vi "PhotonPoseEstimator_multiTagOnCoprocStrategy.vi"(10 "CameraResult":T11, 11 "PhotonPoseEstimator_REF":T1) -> (0 "Do Alt Strategy":bool, 1 "Pos Found":bool, 3 "PhotonEstimatedRobotPose":T2={"EstimatedPose"={"Translation3d"={"X"=0.0, "Y"=0.0, "Z"=0.0}, "Rotation3d"={"Q_quaternion"={"R"=1.0, "V"=[0.0, 0.0, 0.0]}}}, "TimeStamp_Seconds"=0.0, "targetsUsed"=[], "Strategy"=enum."LOWEST_AMBIGUITY"} {"targetsUsed"."AltCameraToTarget"."TRANSLATION3D"."Z" format="%14.3f"; "targetsUsed"."AltCameraToTarget"."TRANSLATION3D"."Y" format="%14.3f"; "targetsUsed"."AltCameraToTarget"."TRANSLATION3D"."X" format="%14.3f"; "targetsUsed"."BestCameraToTarget"."TRANSLATION3D"."Z" format="%14.3f"; "targetsUsed"."BestCameraToTarget"."TRANSLATION3D"."Y" format="%14.3f"; "targetsUsed"."BestCameraToTarget"."TRANSLATION3D"."X" format="%14.3f"; "EstimatedPose"."Translation3d"."Z" format="%14.3f"; "EstimatedPose"."Translation3d"."Y" format="%14.3f"; "EstimatedPose"."Translation3d"."X" format="%14.3f"})   [LabVIEW 2019, in "PhotonVisionLib.lvlib"]
doc: "This is an internal function. Use Update or Update_Pipeline instead of this function.\n\nDetermine the best target based the multi-target routine on the coprocessor"
uses:
  PhotonVisionLib.lvlib
  Enum/PhotonPoseStrategy_ENUM.ctl
  <vilib>/Rock Robotics/WPI/ThirdParty/JAS_Junk/TrajLib/Trajectory_Library.lvlib
  <vilib>/Rock Robotics/WPI/ThirdParty/JAS_Junk/TrajLib/TypeDef/TRANSLATION3D.ctl
  <vilib>/Rock Robotics/WPI/ThirdParty/JAS_Junk/TrajLib/TypeDef/QUATERNION.ctl
  <vilib>/Rock Robotics/WPI/ThirdParty/JAS_Junk/TrajLib/TypeDef/ROTATION3D.ctl
  <vilib>/Rock Robotics/WPI/ThirdParty/JAS_Junk/TrajLib/TypeDef/TRANSFORM3D.ctl
  <vilib>/Rock Robotics/WPI/ThirdParty/JAS_Junk/TrajLib/TypeDef/POSE3D.ctl
  TypeDef/PhotonEstimatedRobotPoseType.ctl
  TypeDef/TargetCornerType.ctl
  TypeDef/PhotonTrackedTargetType.ctl
  TypeDef/PhotonPipelineResultType.ctl
  <vilib>/Rock Robotics/WPI/ThirdParty/JAS_Junk/TrajLib/TypeDef/AprilTag.ctl
  <vilib>/Rock Robotics/WPI/ThirdParty/JAS_Junk/TrajLib/Enum/AprilTagFieldLayoutOrignPosition_ENUM.ctl
  <vilib>/Rock Robotics/WPI/ThirdParty/JAS_Junk/TrajLib/TypeDef/AprilTagFieldLayout.ctl
  TypeDef/PhotonPoseEstimatorType.ctl
  TypeDef/PhotonPNPResultType.ctl
  TypeDef/PhotonMultiTargetPNPResultType.ctl
  TypeDef/PhotonTargetModel.ctl
  Ref/PhotonPipelineResult_REF.ctl
  Ref/PhotonPoseEstimator_REF.ctl
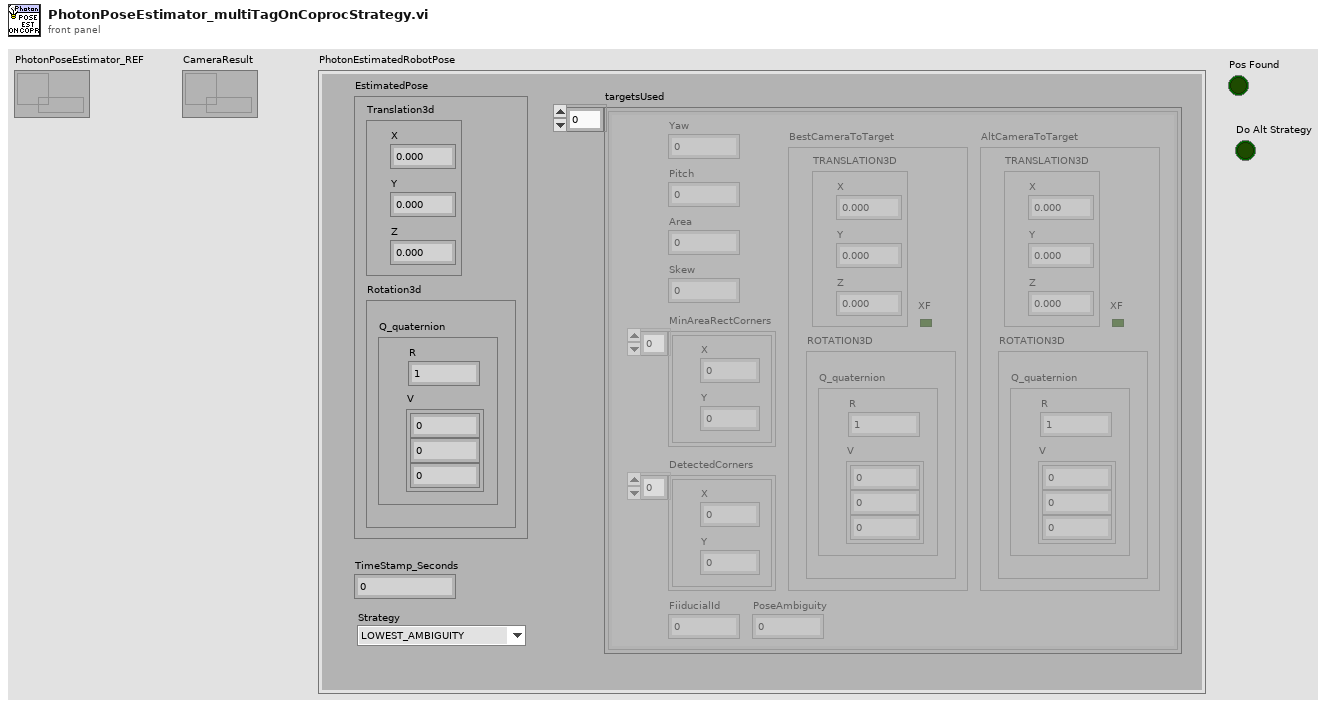
[diagram p1: front panel]
types:
  T1 = typedef "PhotonVisionLib.lvlib/PhotonPoseEstimator_REF.ctl" = refnum<data-value>
  T2 = typedef "PhotonVisionLib.lvlib/PhotonEstimatedRobotPoseType.ctl" = cluster{"EstimatedPose":T3, "TimeStamp_Seconds":dbl, "targetsUsed":T7[], "Strategy":T10}
  T3 = typedef "Trajectory_Library.lvlib/POSE3D.ctl" = cluster{"Translation3d":T4, "Rotation3d":T5}
  T4 = typedef "Trajectory_Library.lvlib/TRANSLATION3D.ctl" = cluster{"X":dbl, "Y":dbl, "Z":dbl}
  T5 = typedef "Trajectory_Library.lvlib/ROTATION3D.ctl" = cluster{"Q_quaternion":T6}
  T6 = typedef "Trajectory_Library.lvlib/QUATERNION.ctl" = cluster{"R":dbl, "V":dbl[]}
  T7 = typedef "PhotonVisionLib.lvlib/PhotonTrackedTargetType.ctl" = cluster{"Yaw":dbl, "Pitch":dbl, "Area":dbl, "Skew":dbl, "MinAreaRectCorners":T8[], "BestCameraToTarget":T9, "FiiducialId":i32, "AltCameraToTarget":T9, "PoseAmbiguity":dbl, "DetectedCorners":T8[]}
  T8 = typedef "PhotonVisionLib.lvlib/TargetCornerType.ctl" = cluster{"X":dbl, "Y":dbl}
  T9 = typedef "Trajectory_Library.lvlib/TRANSFORM3D.ctl" = cluster{"TRANSLATION3D":T4, "ROTATION3D":T5, "XF":bool}
  T10 = typedef "PhotonVisionLib.lvlib/PhotonPoseStrategy_ENUM.ctl" = enum16{"LOWEST_AMBIGUITY", "CLOSEST_TO_CAMERA_HEIGHT", "CLOSEST_TO_REFERENCE_POSE", "CLOSEST_TO_LAST_POSE", "AVERAGE_BEST_TARGETS", "MULTI_TAG_PNP_ON_COPROCESSOR", "MULTI_TAG_PNP_ON_RIO"}
  T11 = typedef "PhotonVisionLib.lvlib/PhotonPipelineResult_REF.ctl" = refnum<data-value>
  T12 = typedef "PhotonVisionLib.lvlib/PhotonMultiTargetPNPResultType.ctl" = cluster{"PhotonPNPResult":T13, "FiducialIDsUsed":i16[]}
  T13 = typedef "PhotonVisionLib.lvlib/PhotonPNPResultType.ctl" = cluster{"IsPresent":bool, "bestReprojErr":dbl, "altReprojErr":dbl, "ambiguity":dbl, "Best":T9, "Alt":T9}
  T14 = typedef "Trajectory_Library.lvlib/AprilTagFieldLayout.ctl" = cluster{"AprilTagMap":map{i32, T15}, "FieldLength":dbl, "FieldWidth":dbl, "OriginPosition ":T16, "OriginPose3d":T3}
  T15 = typedef "Trajectory_Library.lvlib/AprilTag.ctl" = cluster{"ID":i32, "POSE3D":T3}
  T16 = typedef "Trajectory_Library.lvlib/AprilTagFieldLayoutOrignPosition_ENUM.ctl" = enum16{"kBlueAllianceWallRightSide,", "kRedAllianceWallRightSide,"}
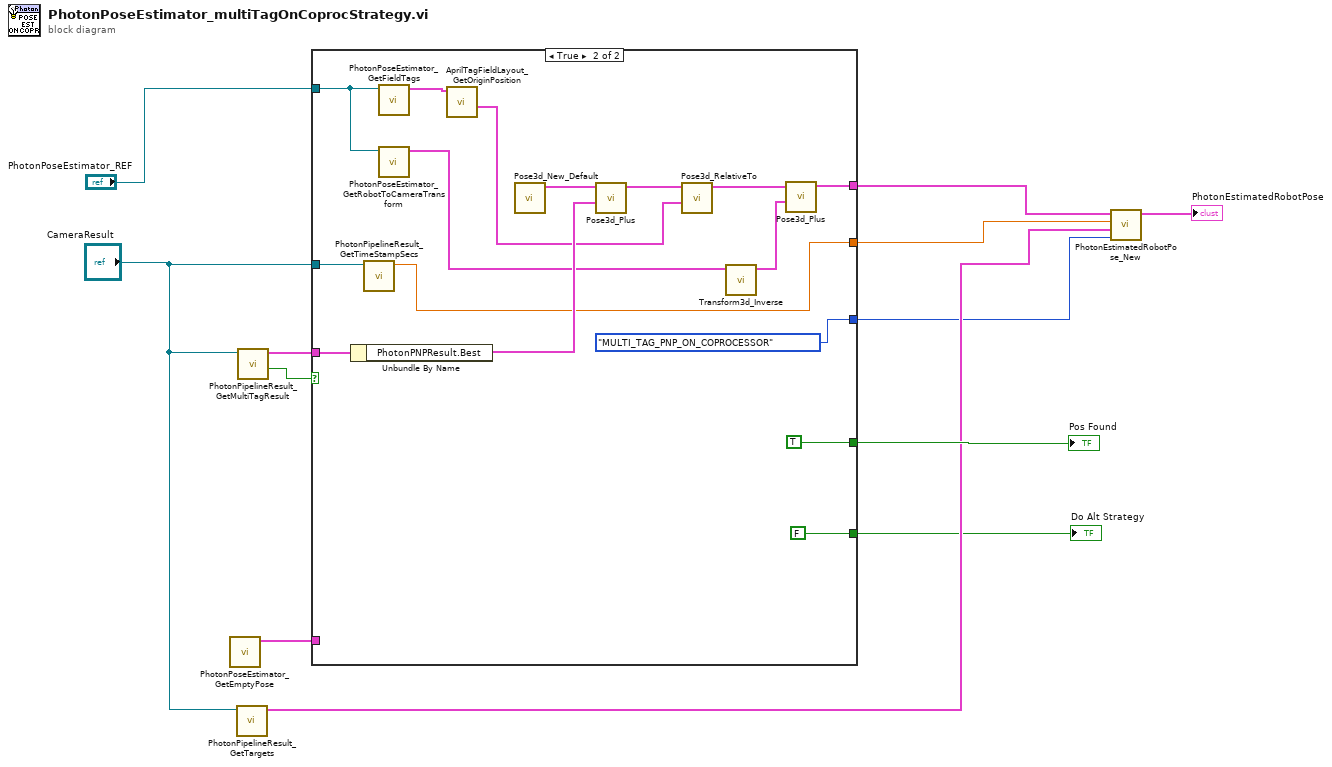
[diagram p0: block diagram]
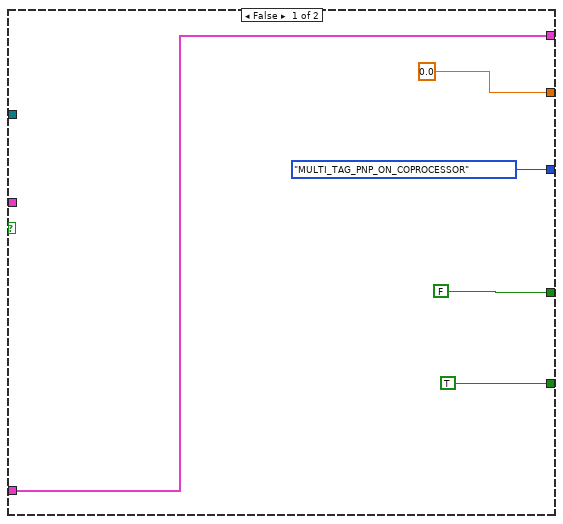
[diagram p2: hidden frame]
diagram:
  n1 = call "PhotonPoseEstimator_GetEmptyPose.vi"() -> ("EmptyPose"=w11:T3)  [unwired: 11 in]
  n2 = call "PhotonPipelineResult_GetTargets.vi"("PhotonPipelineResult_REF"="CameraResult") -> ("Targets"=w6:T7[])  [unwired: 10 in]
  n3 = call "PhotonPipelineResult_GetMultiTagResult.vi"("PhotonPipelineResult_REF"="CameraResult") -> ("Is Present"=w4:bool, "PhotonMultiTargetPNPResult"=w3:T12)  [unwired: 9 in]
  n4 = case shown="True" w4 {
    tunnel: "CameraResult" -> [_ w18]
    tunnel: [FALSE ("Found") TRUE ("Found")] -> w12
    tunnel: "PhotonPoseEstimator_REF" -> [_ w19]
    tunnel: w11 -> [w16 _]
    tunnel: [0.0 ("TimeStamp_Seconds") w20] -> w9
    tunnel: [w16 w24] -> w8
    tunnel: w3 -> [_ w33]
    tunnel: [PhotonPoseStrategy_ENUM."MULTI_TAG_PNP_ON_COPROCESSOR" ("Strategy") PhotonPoseStrategy_ENUM."MULTI_TAG_PNP_ON_COPROCESSOR" ("Strategy")] -> w2
    tunnel: [TRUE ("Found") FALSE ("Found")] -> w1
    frame False {
    }
    frame True {
      n5 = Unbundle By Name(w33) -> ("PhotonPNPResult.Best"=w31:T9)
      n6 = call "PhotonPipelineResult_GetTimeStampSecs.vi"("PhotonPipelineResult_REF"=w18) -> ("TimeStampSec"=w20:dbl)  [unwired: 10 in]
      n7 = call "PhotonPoseEstimator_GetFieldTags.vi"("PhotonPoseEstimator"=w19) -> ("AprilTagFieldLayout"=w29:T14)  [unwired: 10 in]
      n8 = call "PhotonPoseEstimator_GetRobotToCameraTransform.vi"("PhotonPoseEstimator"=w19) -> ("RobotToCamera"=w25:T9)  [unwired: 10 in]
      n9 = call <vilib>:"AprilTagFieldLayout_GetOriginPosition.vi"("AprilTagFieldLayout"=w29) -> ("OriginPose3d"=w28:T3)  [unwired: 9 in, 1 out]
      n10 = call <vilib>:"Pose3d_New_Default.vi"() -> ("outPose3d"=w32:T3)  [unwired: 11 in]
      n11 = call <vilib>:"Pose3d_Plus.vi"("other Transform3d"=w31, "in Pose3d"=w32) -> ("out Pose3d"=w30:T3)  [unwired: 9 in]
      n12 = call <vilib>:"Pose3d_RelativeTo.vi"("other Pose3d"=w28, "in Pose3d"=w30) -> ("out Pose3d"=w27:T3)  [unwired: 9 in]
      n13 = call <vilib>:"Transform3d_Inverse.vi"("inTransform3d"=w25) -> ("outTransform3d"=w26:T9)  [unwired: 10 in]
      n14 = call <vilib>:"Pose3d_Plus.vi"("other Transform3d"=w26, "in Pose3d"=w27) -> ("out Pose3d"=w24:T3)  [unwired: 9 in]
    }
  }
  "Pos Found" <- w12
  "Do Alt Strategy" <- w1
  n15 = call "PhotonEstimatedRobotPose_New.vi"("Strategy"=w2, "targetsUsed"=w6, "TimeStamp_Seconds"=w9, "EstimatedPose"=w8) -> ("PhotonEstimatedRobotPose"=→"PhotonEstimatedRobotPose":T2)  [unwired: 7 in]
